vi "1B_FindOffsetStart.vi"(0 "waveform":waveform(dbl), 1 "Smoothing Strength":T1=enum."10") -> (2 "floor Length":dbl, 3 "start of floor index":dbl)   [LabVIEW 2010]
uses:
  FilterStrength.ctl
  <vilib>/measure/mamon.llb/Waveform Peak Detection for 1 Chan.vi
  <vilib>/measure/NI_MAPro.lvlib
panel:
  in  "Draw":bool
  out "max index":i32
  out "last peak or valley index":dbl
  out "last valley time":dbl
  out "last peak time":dbl
  out "XY Graph":cluster{dbl[], dbl[]}[](graph)
  out "# peaks found":i32
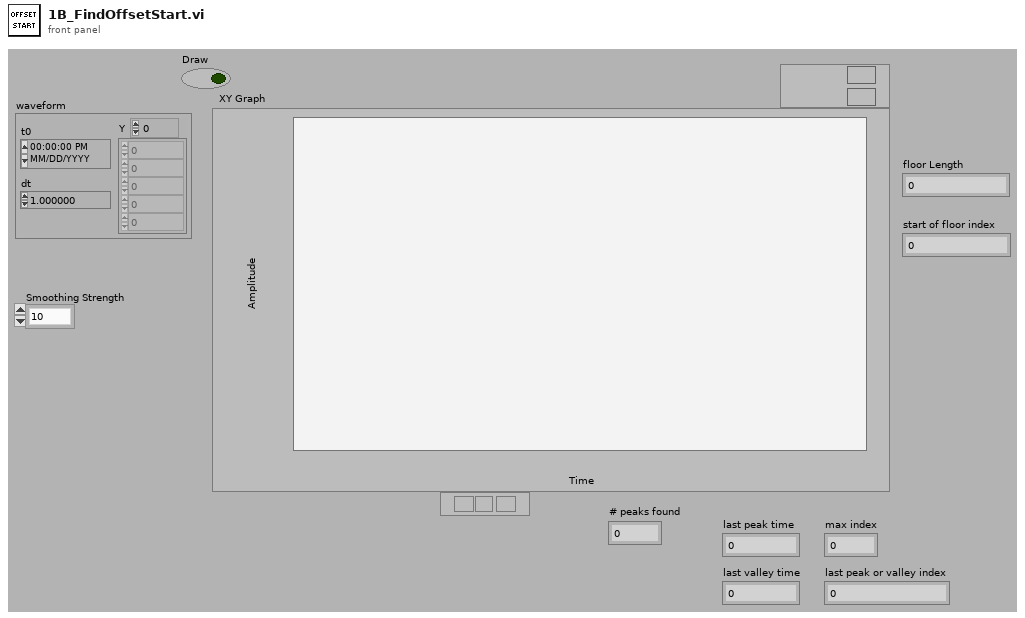
[diagram p1: front panel]
types:
  T1 = typedef "FilterStrength.ctl" = enum16{"Off", "10", "20", "50", "100", "200", "500", "1000"}
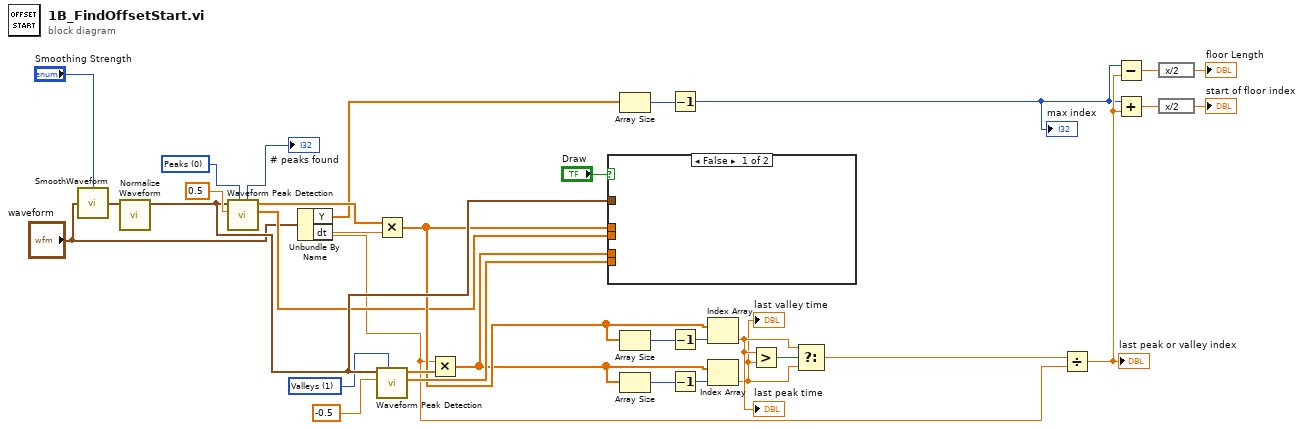
[diagram p0: block diagram]
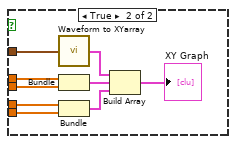
[diagram p2: hidden frame]
diagram:
  w28 = u16 1 items=["Peaks", "Valleys"] ("peaks/valleys")
  w33 = u16 0 items=["Peaks", "Valleys"] ("peaks/valleys")
  n1 = call "SmoothWaveform.vi"("Waveform"="waveform", "Smoothing Strength"="Smoothing Strength") -> ("Filtered data"=w4:waveform(dbl))
  n2 = call <vilib>:"Normalize Waveform.vi"("waveform in"=w4) -> ("normalized waveform"=w29:waveform(dbl))  [unwired: 7 in, 3 out]
  n3 = call-poly <vilib>:"Waveform Peak Detection.vi"("peaks/valleys"=w33, "threshold"=0.5, "Signal In"=w29) -> ("Amplitudes"=w17:dbl[], "Locations"=w30:dbl[], "# found"=→"# peaks found":i32)  [unwired: 4 in, 2 out]
  n4 = Unbundle By Name("waveform") -> ("Y"=w12:dbl[], "dt"=w5:dbl)
  n5 = Multiply(x=w30, y=w5) -> (x*y=w23:dbl[])
  n6 = call-poly <vilib>:"Waveform Peak Detection.vi"("peaks/valleys"=w28, "threshold"=-0.5, "Signal In"=w29) -> ("Amplitudes"=w25:dbl[], "Locations"=w26:dbl[])  [unwired: 4 in, 3 out]
  n7 = Multiply(x=w5, y=w26) -> (x*y=w20:dbl[])
  n8 = case shown="False" "Draw" {
    tunnel: w29 -> [_ w40]
    tunnel: w25 -> [_ w38]
    tunnel: w23 -> [_ w37]
    tunnel: w20 -> [_ w36]
    tunnel: w17 -> [_ w35]
    frame False {
    }
    frame True {
      n9 = call "Waveform to XYarray.vi"("Waveform In"=w40) -> ("Single Plot"=w42:cluster{"X array":dbl[], "Y array":dbl[]})
      n10 = Bundle(w37, "Amplitudes"=w35) -> (w41:cluster{dbl[], "Amplitudes":dbl[]})  [unwired: 1 in]
      n11 = Bundle(w36, "Amplitudes"=w38) -> (w39:cluster{dbl[], "Amplitudes":dbl[]})  [unwired: 1 in]
      n12 = Build Array(w42, w41, w39) -> (→"XY Graph":cluster{"X array":dbl[], "Amplitudes":dbl[]}[])
    }
  }
  n13 = Array Size(array=w12) -> (size(s)=w13:i32)
  n14 = Array Size(array=w23) -> (size(s)=w24:i32)
  n15 = Array Size(array=w20) -> (size(s)=w22:i32)
  n16 = Decrement(x=w13) -> (x-1=w7:i32)
  "max index" <- w7
  n17 = Decrement(x=w24) -> (x-1=w18:i32)
  n18 = Decrement(x=w22) -> (x-1=w21:i32)
  n19 = Index Array(array=w23, index=w18) -> (element=w16:dbl)
  "last peak time" <- w16
  n20 = Index Array(array=w20, index=w21) -> (element=w15:dbl)
  "last valley time" <- w15
  n21 = Greater?(x=w16, y=w15) -> (0:w19:bool)
  n22 = Select(t=w16, s=w19, f=w15) -> (s? t:f=w14:dbl)
  n23 = Divide(x=w14, y=w5) -> (x/y=w11:dbl)
  "last peak or valley index" <- w11
  n24 = Subtract(x=w7, y=w11) -> (x-y=w9:dbl)
  n25 = Add(x=w7, y=w11) -> (x+y=w10:dbl)
  n26 = expression code="x/2"(w9) -> (→"floor Length":dbl)
  n27 = expression code="x/2"(w10) -> (→"start of floor index":dbl)
